vi "Simple Reader.vi"(8 "error in (no error)":errorcluster, 11 "Oxford PS Driver in":refnum<class "Oxford PS Driver.lvclass">) -> (0 "error out":errorcluster, 2 "Signals":dbl[](array[numeric]), 3 "Oxford PS Driver out":refnum<class "Oxford PS Driver.lvclass">)   [LabVIEW 2016, in "Oxford PS Driver.lvclass"]
uses:
  Oxford PS Driver.lvclass
  C:/github/NHMFL_Core/Libraries/Instruments/VISA Instrument/VISA Instrument.lvclass
  VISA Instrument/VISA Instrument.lvclass/VISA Instrument.ctl
  VISA Instrument/Read VISA resource.vi
  VISA Instrument/Write VISA resource.vi
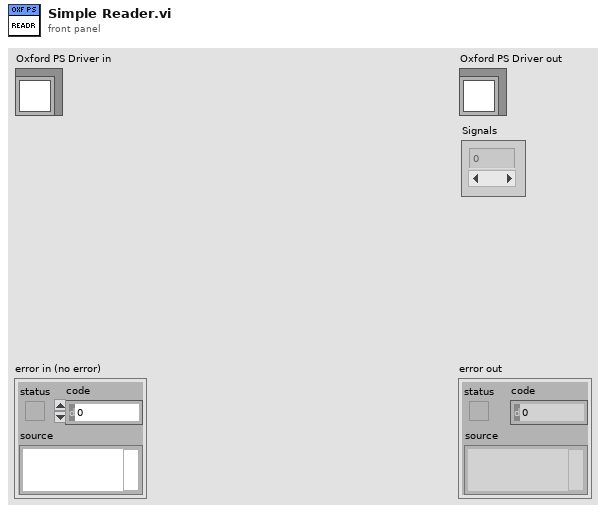
[diagram p1: front panel]
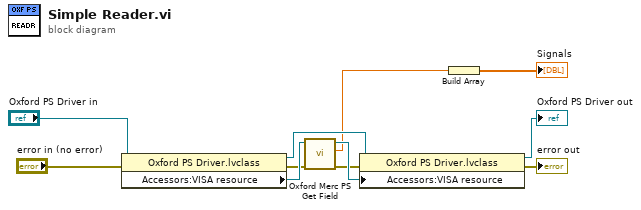
[diagram p0: block diagram]
diagram:
  n1 = property class="Oxford PS Driver.lvclass"(reference="Oxford PS Driver in", error in="error in (no error)") -> (reference out=w7:refnum<class "Oxford PS Driver.lvclass">, error out=w8:errorcluster, "Accessors:VISA resource"=w11:refnum<visa-resource-name>)
  n2 = call "Oxford Merc PS Get Field.vi"("Error In"=w8, "VISA resource name"=w11) -> ("Error Out"=w1:errorcluster, "Magnetic Field (T)"=w4:dbl, "VISA resource name out"=w6:refnum<visa-resource-name>)  [unwired: 7 in]
  n3 = property class="Oxford PS Driver.lvclass"(reference=w7, error in=w1, "Accessors:VISA resource"=w6) -> (reference out=→"Oxford PS Driver out":refnum<class "Oxford PS Driver.lvclass">, error out=→"error out":errorcluster)
  n4 = Build Array(w4) -> (→"Signals":dbl[])
